vi "Process.vi"(8 "error in (no error)":errorcluster, 11 "DB2":refnum<class "DB2.lvclass">) -> (0 "error out":errorcluster, 3 "DB2 out":refnum<class "DB2.lvclass">)   [LabVIEW 2022 SP3, in "DB2.lvclass"]
uses:
  DB2.lvclass
  C:/Program Files (x86)/National Instruments/LabVIEW 2022/vi.lib/JKI/JKI SMO/SMO/SMO.lvclass
  <vilib>/JKI/JKI SMO/SMO/Typedefs/Parent Call--Enum.ctl
  Typedefs/PublicEvents--DB2.NewSettingsConfig.ctl
  <vilib>/JKI/JKI SMO/SMO/SMO.lvclass
  <vilib>/JKI/JKI SMO/SMO/SMO.lvclass/SMO.ctl
  <vilib>/JKI/JKI SMO/SMO/Private/GetVariant(Attr).vi
  <vilib>/JKI/JKI SMO/Support/Attribute.Identity/Read UniqueName.vi
  <vilib>/JKI/JKI SMO/Support/Attribute.Identity/Read Given Name.vi
  <vilib>/JKI/JKI SMO/Support/Attribute.Identity/Read ProspectiveOwner.vi
  <vilib>/JKI/JKI SMO/SMO/Private/ReftoDVR--SMO.vi
  <vilib>/JKI/JKI SMO/Support/Attribute.Identity/Attribute.Identity.lvclass
panel:
  in  "Cancel Button":bool
  in  "Save Button":bool
  in  "Source Code to Analyze":path
  in  "Report Generation Save Path":path
  in  "Requirements Definition (.csv)":path
  in  "OK":bool
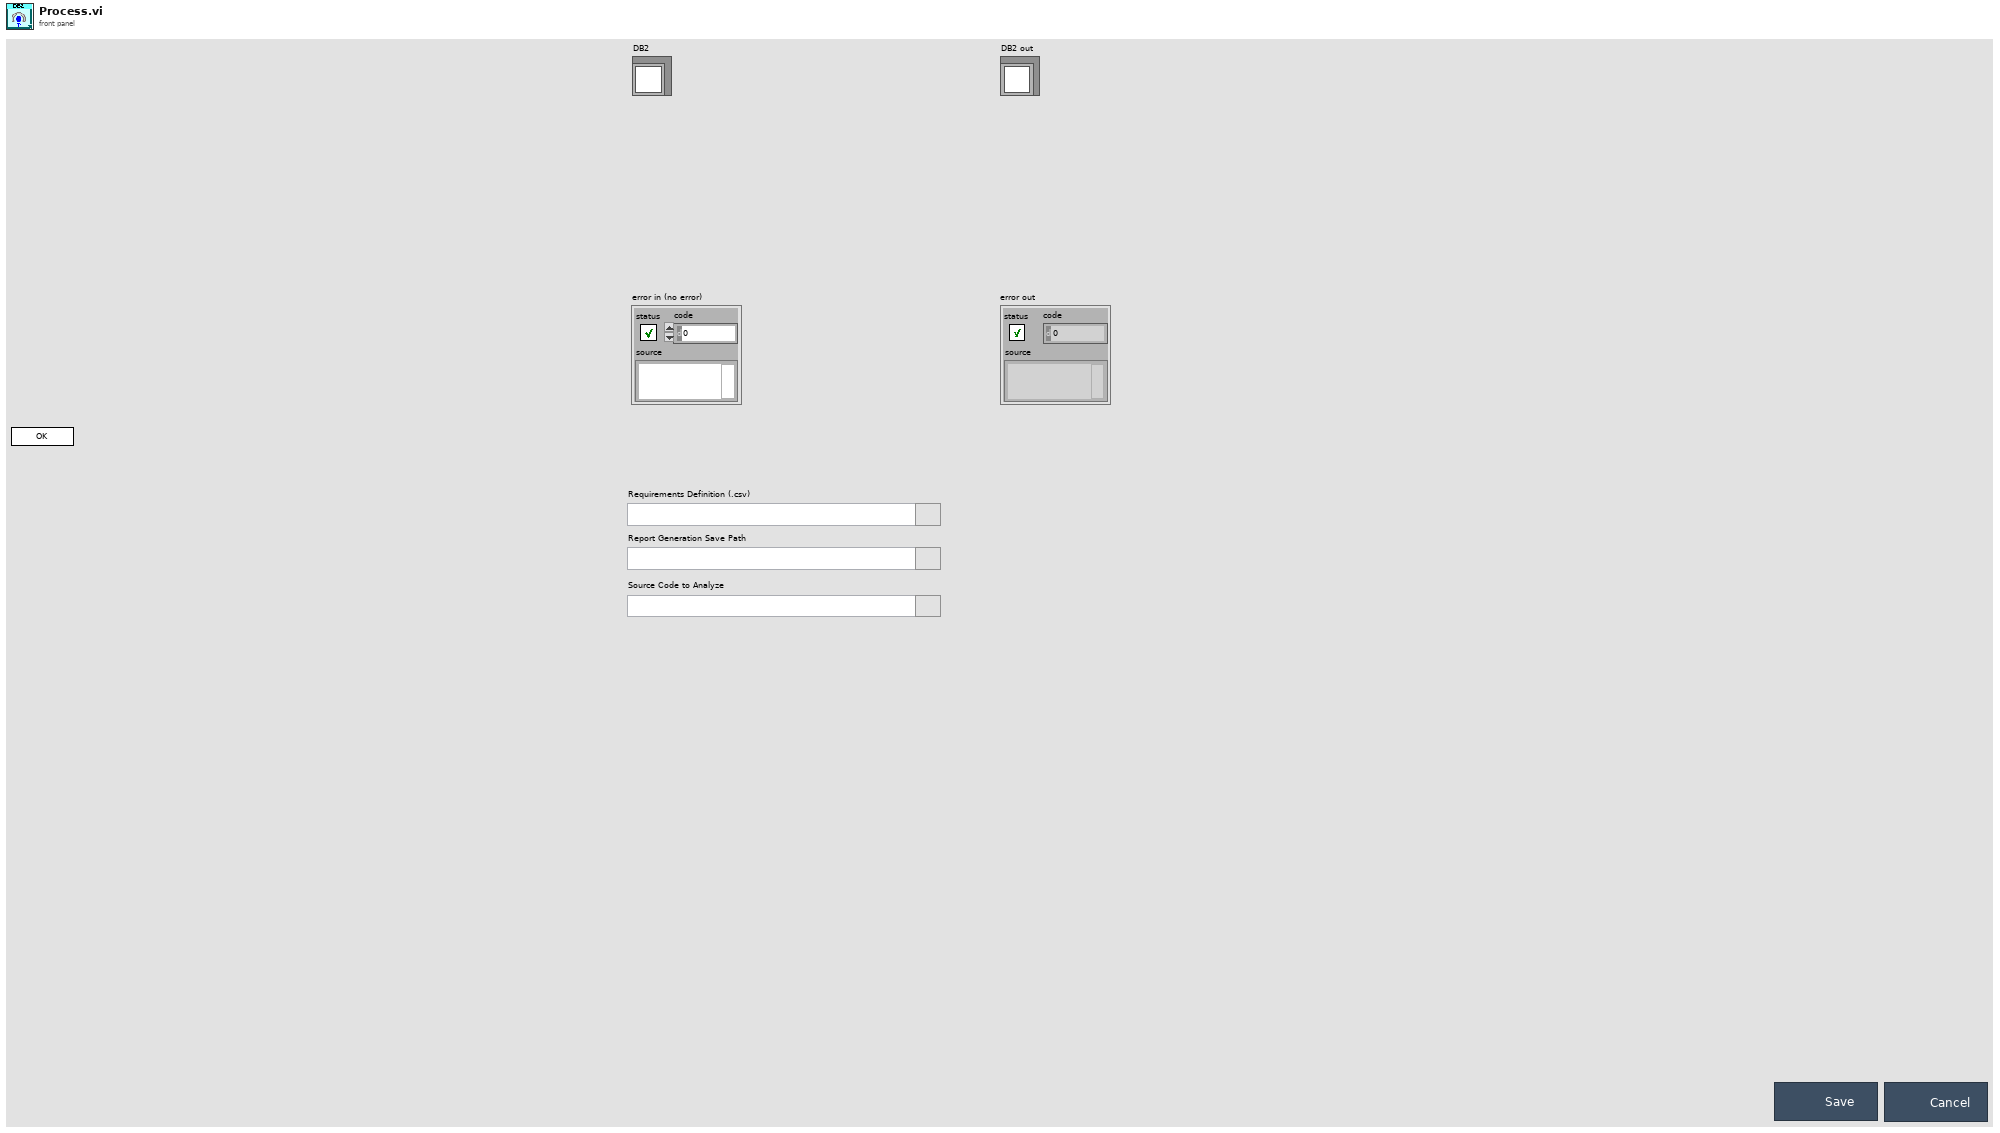
[diagram p1: front panel]
types:
  T1 = typedef "SMO.lvclass/Parent Call--Enum.ctl" = enum16{"Allows parent to run", "Does not request parent to run"}
  T2 = typedef "DB2.lvclass/PublicEvents--DB2.NewSettingsConfig.ctl" = cluster{"Requirements Definition (.csv)":path, "Report Generation Save Path":path, "Source Code to Analyze":path, "Search By:":string, "Word/Phrase:":string}
  T3 = enum32{"invalid app kind", "Development System", "Run Time System", "Student Edition", "Embedded LabVIEW", "Evaluation", "Custom"}
  T4 = enum32{"Invalid", "Standard", "Closed", "Hidden", "Minimized", "Maximized"}
  T5 = typedef "DB2.lvclass/DB2 State--enum.ctl" = enum16{"unknown", "Opened", "Embedded", "Closed"}
  T6 = cluster{"Core":cluster{"Current VI Reference":refnum<vi>, "Close Panel on Exit?":bool, "error":errorcluster}, "Self Ref":refnum<class "DB2.lvclass">, "New Settings Config":T2}
  T7 = cluster{"Current VI Reference":refnum<vi>, "Close Panel on Exit?":bool, "error":errorcluster}
  T8 = typedef "SMO.lvclass/Protected Events.ctl" = cluster{"StopProcesses":refnum<user-event>, "AbortProcesses":refnum<user-event>, "Config Changed":refnum<user-event>, "Dependency":refnum<user-event>}
  T9 = typedef "DB2.lvclass/PublicEvents--Cluster.ctl" = cluster{"UI State":refnum<user-event>, "NewSettingsConfig":refnum<user-event>}
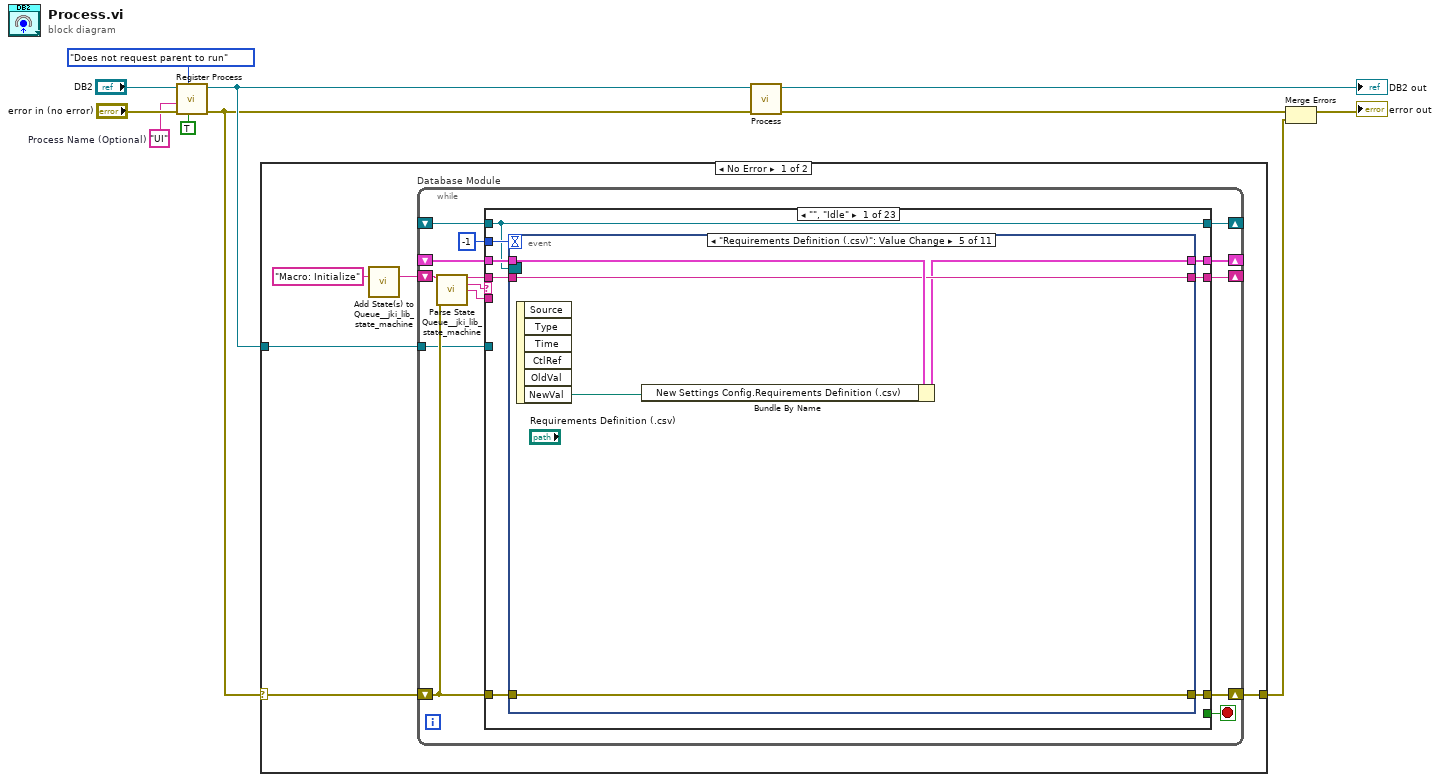
[diagram p0: block diagram]
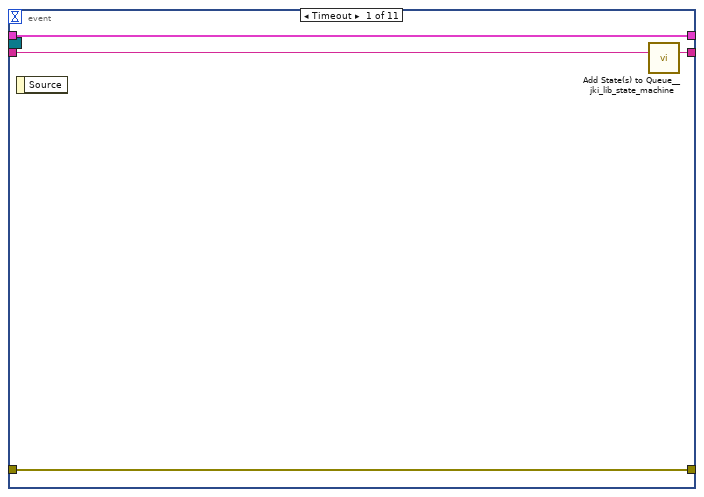
[diagram p2: hidden frame]
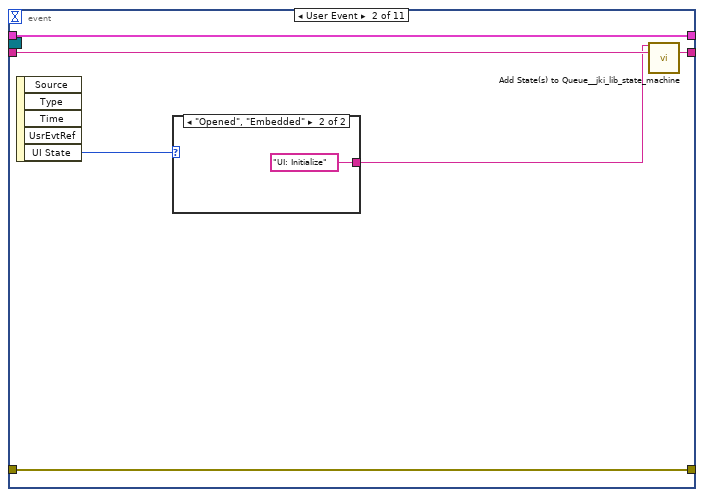
[diagram p3: hidden frame]
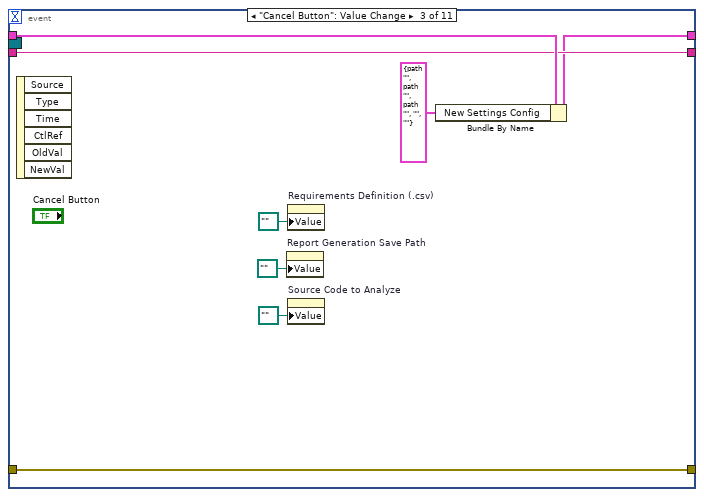
[diagram p5: hidden frame]
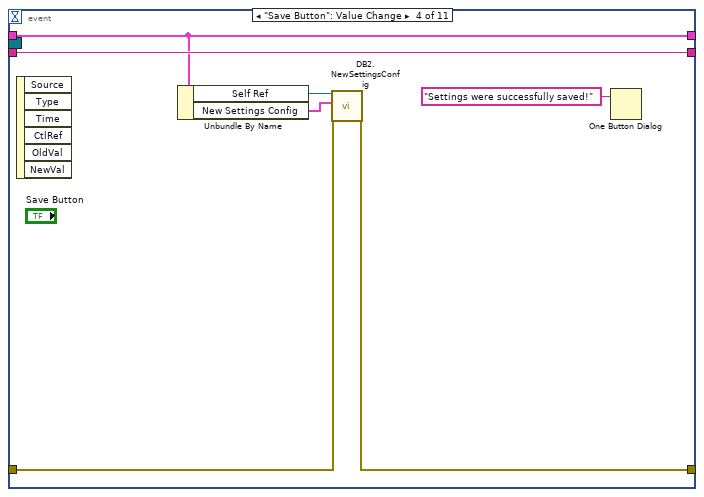
[diagram p6: hidden frame]
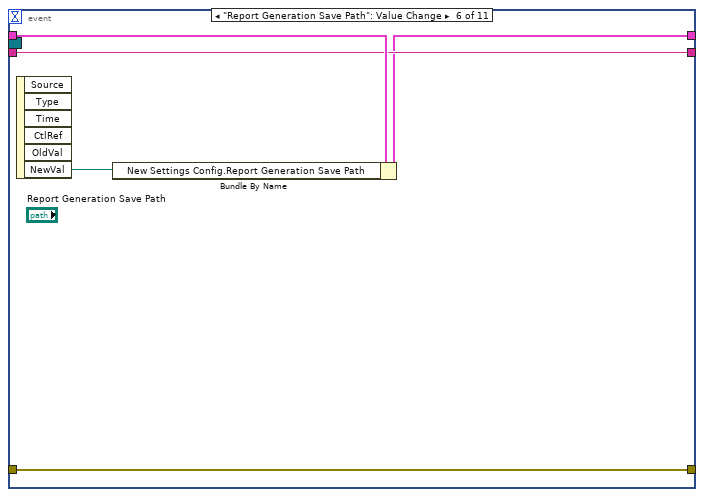
[diagram p7: hidden frame]
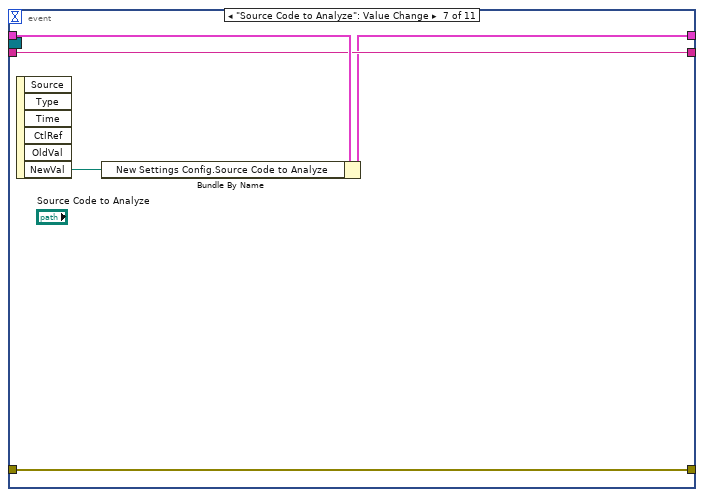
[diagram p8: hidden frame]
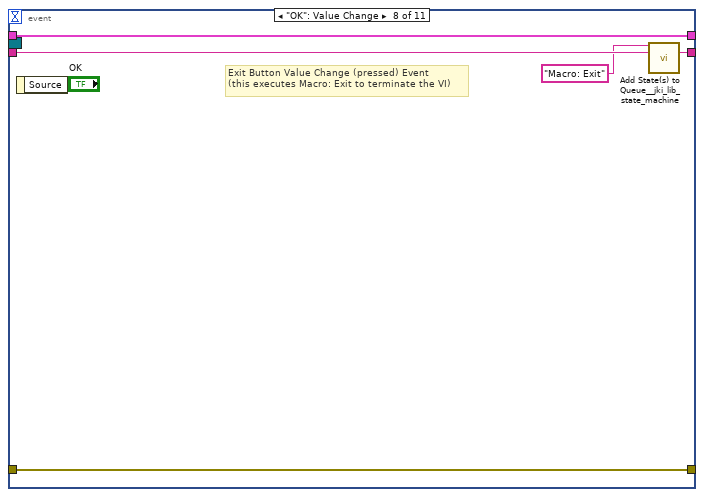
[diagram p9: hidden frame]
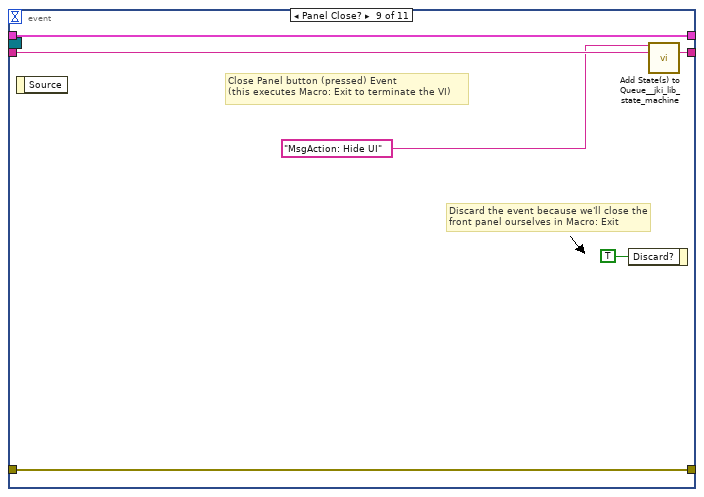
[diagram p10: hidden frame]
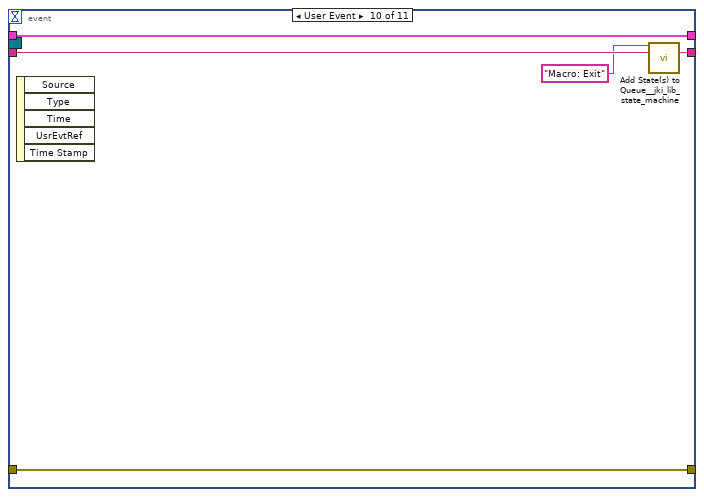
[diagram p11: hidden frame]
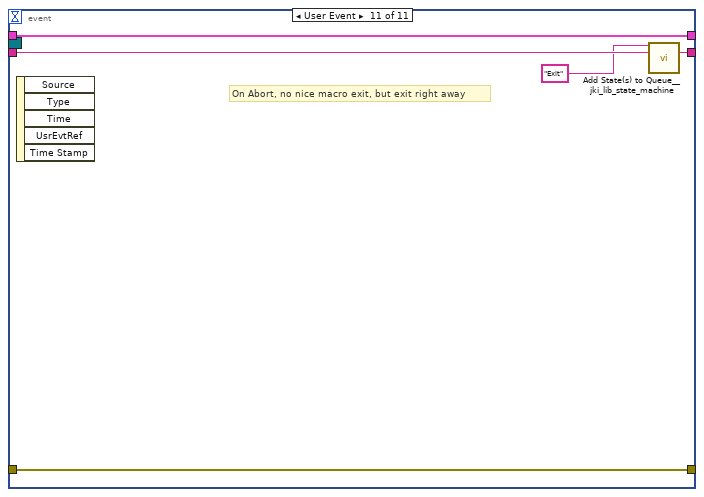
[diagram p12: hidden frame]
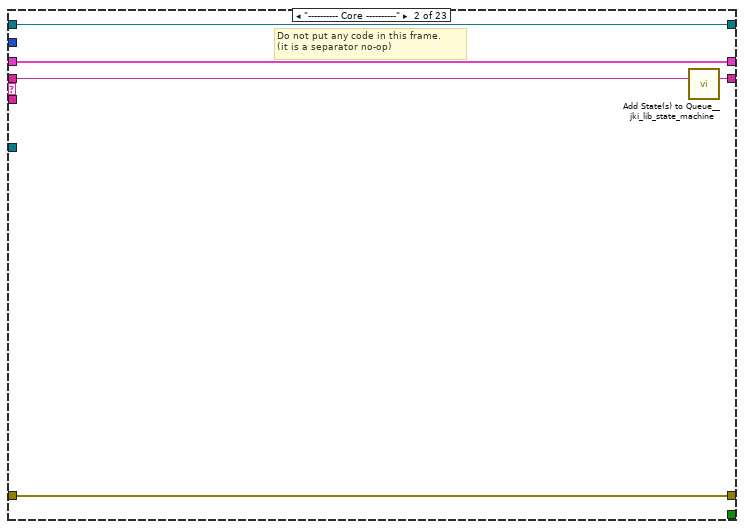
[diagram p13: hidden frame]
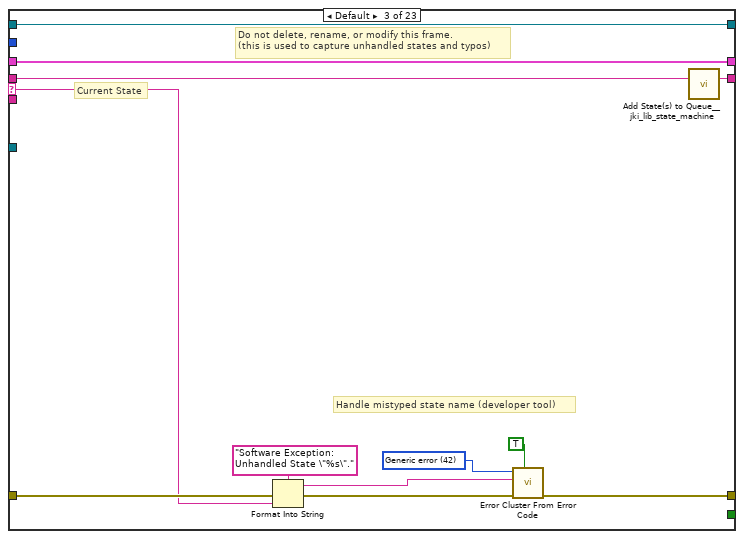
[diagram p14: hidden frame]
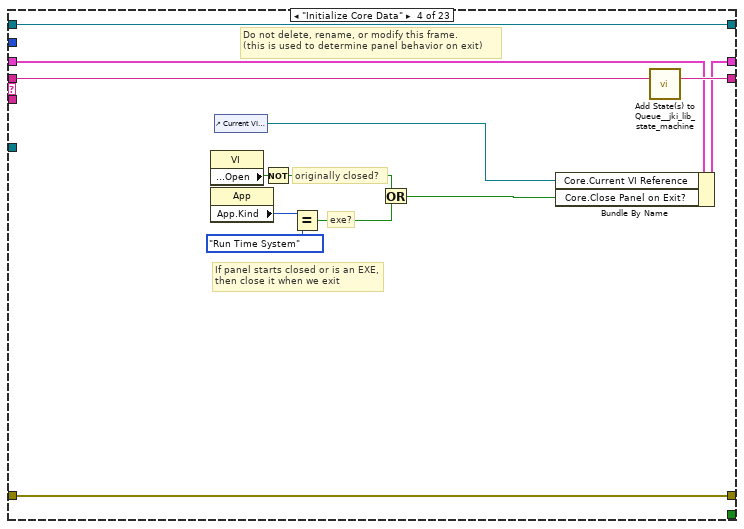
[diagram p15: hidden frame]
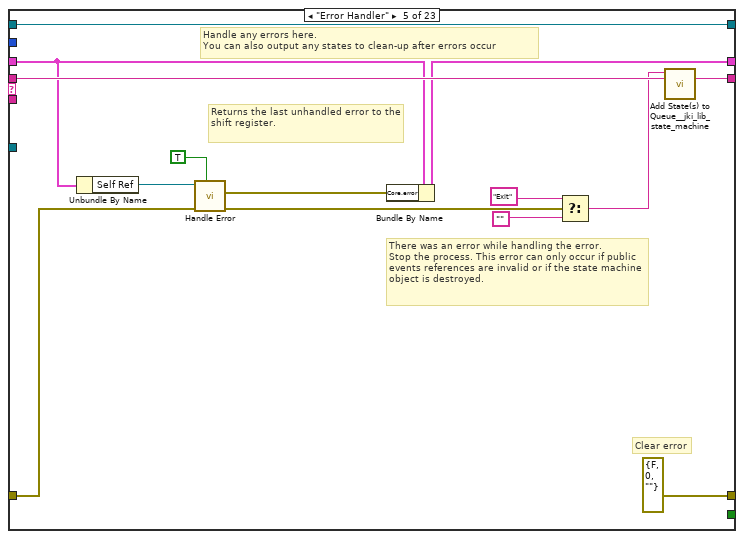
[diagram p16: hidden frame]
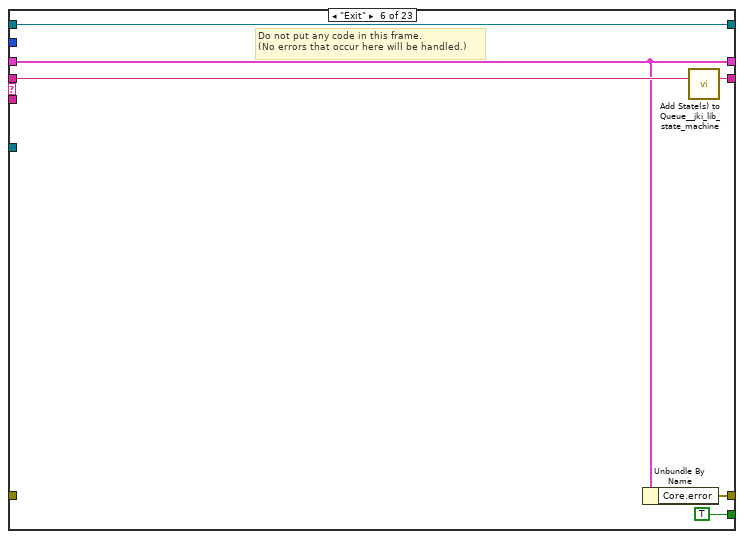
[diagram p17: hidden frame]
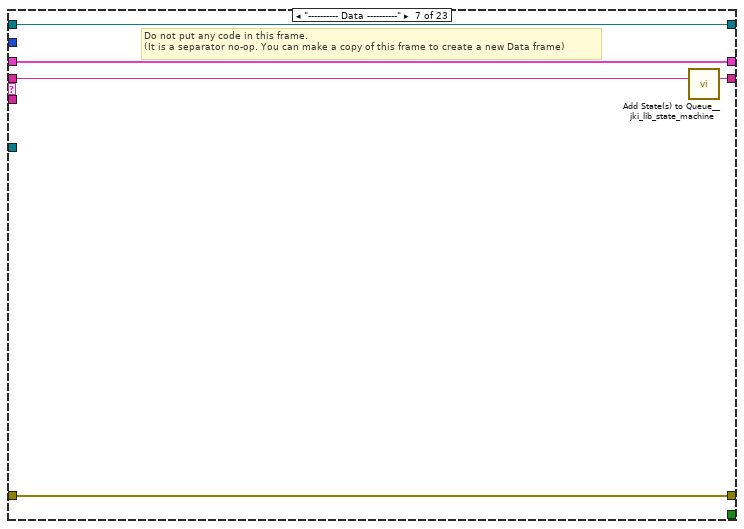
[diagram p18: hidden frame]
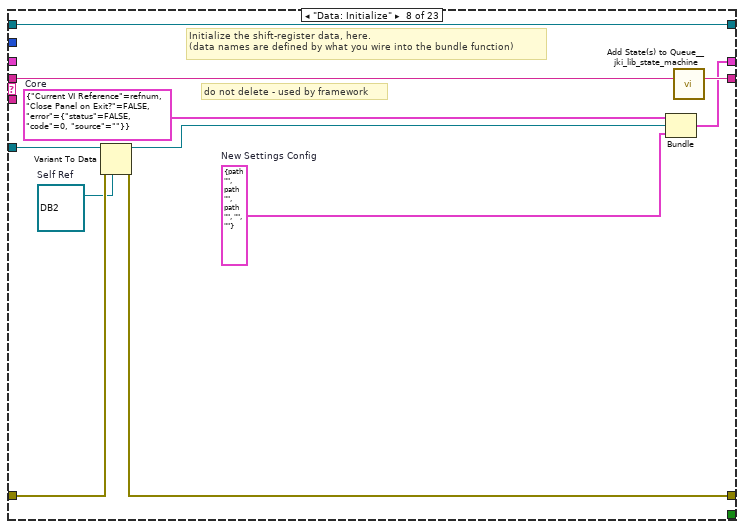
[diagram p19: hidden frame]
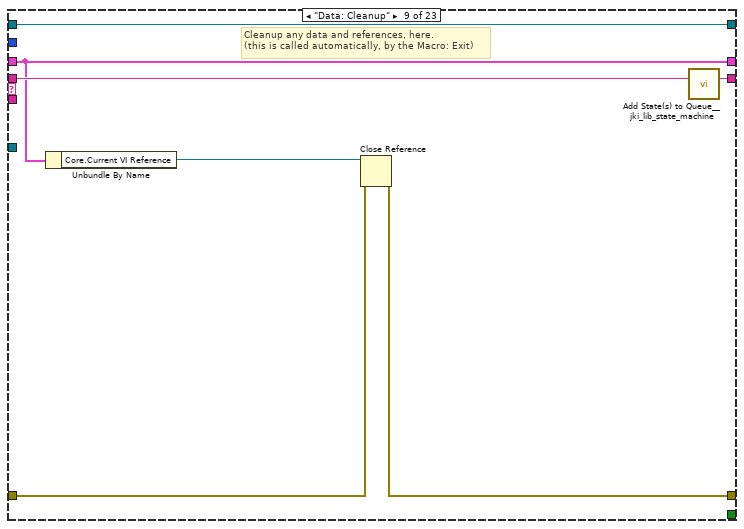
[diagram p20: hidden frame]
diagram:
  w4 = "UI"  # Process Name (Optional)
  n1 = call <vilib>:"Register Process.vi"("Forces Self to Run (F)"=TRUE, "Parent Call"=Parent_Call--Enum."Does not request parent to run", "error in (no error)"="error in (no error)", "Process Name (optional)"=w4, "SMO"="DB2") -> ("error out"=w10:errorcluster, "SMO out"=w11:refnum<class "DB2.lvclass">)  [unwired: 5 in]
  n2 = case shown="No Error" w10 {
    selector: w10 -> [w13 w318]
    tunnel: w11 -> [w14 _]
    tunnel: [w12 w318] -> w8
    frame No Error {
      n3 = call <vilib>:"Add State(s) to Queue__jki_lib_state_machine.vi"("State(s) in (\"\")"="Macro: Initialize") -> ("States Out"=w16:string)  [unwired: 14 in]
      n4 = while "Database Module" {
        shift-right: [w23] -> _
        shift-left: _ -> [w22]
        shift-right: [w26] -> w12
        shift-left: w13 -> [w20]
        shift-right: [w25] -> _
        shift-left: w16 -> [w27]
        tunnel: w14 -> [w19]
        shift-right: [w18] -> _
        shift-left: _ -> [w17]
        stop <- w24 stop-if-true
        n5 = call <vilib>:"Parse State Queue__jki_lib_state_machine.vi"("State Queue"=w27, "Error In (no error)"=w20) -> ("Remaining States"=w29:string, "Current State"=w30:string, "Arguments"=w28:string)  [unwired: 11 in]
        n6 = case shown="\"\", \"Idle\"" w30 {
          selector: w30 -> [_ _ w107 _ _ _ _ _ _ _ _ _ _ _ _ _ _ _ _ _ _ _ _]
          tunnel: w29 -> [w38 w105 w111 w130 w144 w150 w155 w166 w173 w178 w186 w193 w209 w241 w250 w261 w266 w277 w289 w294 w306 w312 w317]
          tunnel: w28 -> [_ _ _ _ _ _ _ _ _ _ _ w187 w205 _ _ _ _ _ _ _ _ _ _]
          tunnel: w22 -> [w36 w102 w109 w121 w140 w145 w152 _ w168 w175 w184 w191 w207 w238 w246 w252 w263 w274 w286 w291 w304 w310 w314]
          tunnel: [w35 w103 w113 w127 errorcluster {"status"=FALSE, "code"=0, "source"=""} ("error out") w146 w153 w158 w169 w176 w183 w188 w202 w239 w248 w259 w264 w268 w284 w292 w302 w308 w315] -> w26
          tunnel: w20 -> [w34 w103 w112 w127 w137 _ w153 w163 w170 w176 w183 w189 w203 w239 w248 w259 w264 w269 w281 w292 w295 w308 w315]
          tunnel: [w37 w104 w110 w129 w143 w149 w154 w165 w172 w177 w185 w192 w208 w240 w249 w260 w265 w276 w288 w293 w305 w311 w316] -> w25
          tunnel: [_ _ _ _ _ TRUE _ _ _ _ _ _ _ _ _ _ _ _ _ _ _ _ _] -> w24
          tunnel: [w33 w102 w109 w128 w139 w145 w152 w164 w168 w175 w184 w191 w207 w238 w246 w252 w263 w274 w286 w291 w304 w310 w314] -> w23
          tunnel: -1 ("Timeout") -> [w32 _ _ _ _ _ _ _ _ _ _ _ _ _ _ _ _ _ _ _ _ _ _]
          tunnel: w19 -> [_ _ _ _ _ _ _ w162 _ _ _ _ _ _ _ _ _ _ _ _ _ _ _]
          tunnel: [w31 w101 w106 w118 w142 w147 w151 w161 w167 w174 w182 w190 w206 w237 w247 w253 w262 w275 w287 w290 w301 w309 w313] -> w18
          tunnel: w17 -> [w31 w101 w106 w118 w142 w147 w151 w161 w167 w174 w182 w190 w206 w237 w247 w253 w262 w275 w287 w290 _ w309 w313]
          frame "", "Idle" {
            n7 = event shown="[4] \"Requirements Definition (.csv)\": Value Change" {
              selector: w31 -> [_ _ _ _ _ _ _ _ _ _ _]
              dyn-events: _ -> [_ _ _ _ _ _ _ _ _ _ _]
              timeout: w32 -> [_ _ _ _ _ _ _ _ _ _ _]
              tunnel: w38 -> [w42 w48 w56 w64 w68 w73 w78 w84 w90 w95 w100]
              tunnel: [w41 w47 w56 w64 w68 w73 w78 w83 w89 w94 w99] -> w37
              tunnel: w36 -> [w39 w45 w57 w63 w69 w74 w79 w81 w86 w92 w97]
              tunnel: [w40 w46 w55 w59 w67 w72 w77 w82 w88 w93 w98] -> w35
              tunnel: w34 -> [w40 w46 w55 w60 w67 w72 w77 w82 w88 w93 w98]
              tunnel: [w39 w45 w54 w63 w66 w71 w76 w81 w86 w92 w97] -> w33
              event Timeout {
                n8 = event-data() -> ()  [unwired: 1 in, 1 out]
                n9 = call <vilib>:"Add State(s) to Queue__jki_lib_state_machine.vi"("State(s) in (\"\")"=w42) -> ("States Out"=w41:string)  [unwired: 14 in]
              }
              event User Event {
                n10 = event-data() -> ("UI State"=w44:T5)  [unwired: 1 in, 4 out]
                n11 = case shown="\"Opened\", \"Embedded\"" w44 {
                  tunnel: [_ "UI: Initialize" ("State(s) in Front (\"\")")] -> w43
                  frame Default {
                  }
                  frame "Opened", "Embedded" {
                  }
                }
                n12 = call <vilib>:"Add State(s) to Queue__jki_lib_state_machine.vi"("State(s) in Front (\"\")"=w43, "State(s) in (\"\")"=w48) -> ("States Out"=w47:string)  [unwired: 13 in]
              }
              event "Cancel Button": Value Change {
                n13 = event-data() -> ()  [unwired: 1 in, 6 out]
                n14 = property on="Report Generation Save Path" class="Path"("Value"=path "" ("Report Generation Save Path")) -> ()  [unwired: 2 in, 2 out]
                n15 = property on="Requirements Definition (.csv)" class="Path"("Value"=path "" ("Requirements Definition (.csv)")) -> ()  [unwired: 2 in, 2 out]
                n16 = property on="Source Code to Analyze" class="Path"("Value"=path "" ("Source Code to Analyze")) -> ()  [unwired: 2 in, 2 out]
                n17 = Bundle By Name(cluster=w57, "New Settings Config"=T2 {"Requirements Definition (.csv)"=path "", "Report Generation Save Path"=path "", "Source Code to Analyze"=path "", "Search By:"="", "Word/Phrase:"=""}) -> (w54:T6)
              }
              event "Save Button": Value Change {
                n18 = event-data() -> ()  [unwired: 1 in, 6 out]
                n19 = Unbundle By Name(w63) -> ("Self Ref"=w62:refnum<class "DB2.lvclass">, "New Settings Config"=w61:T2)
                n20 = call "DB2.NewSettingsConfig.vi"("error in"=w60, "New Settings Config"=w61, "DB2.lvclass"=w62) -> ("error out"=w59:errorcluster)  [unwired: 7 in, 1 out]
                n21 = One Button Dialog(message="Settings were successfully saved!") -> ()  [unwired: 1 in, 1 out]
              }
              event "Requirements Definition (.csv)": Value Change {
                n22 = event-data() -> ("NewVal"=w65:path)  [unwired: 1 in, 5 out]
                n23 = Bundle By Name(cluster=w69, "New Settings Config.Requirements Definition (.csv)"=w65) -> (w66:T6)
              }
              event "Report Generation Save Path": Value Change {
                n24 = event-data() -> ("NewVal"=w70:path)  [unwired: 1 in, 5 out]
                n25 = Bundle By Name(cluster=w74, "New Settings Config.Report Generation Save Path"=w70) -> (w71:T6)
              }
              event "Source Code to Analyze": Value Change {
                n26 = event-data() -> ("NewVal"=w75:path)  [unwired: 1 in, 5 out]
                n27 = Bundle By Name(cluster=w79, "New Settings Config.Source Code to Analyze"=w75) -> (w76:T6)
              }
              event "OK": Value Change {
                # "Exit Button Value Change (pressed) Event\n(this executes Macro: Exit to terminate the VI)"
                n28 = event-data() -> ()  [unwired: 1 in, 1 out]
                n29 = call <vilib>:"Add State(s) to Queue__jki_lib_state_machine.vi"("State(s) in Front (\"\")"="Macro: Exit", "State(s) in (\"\")"=w84) -> ("States Out"=w83:string)  [unwired: 13 in]
              }
              event Panel Close? {
                # "Discard the event because we'll close the front panel ourselves in Macro: Exit"
                # "Close Panel button (pressed) Event\n(this executes Macro: Exit to terminate the VI)"
                n30 = event-data() -> ()  [unwired: 1 in, 1 out]
                n31 = event-data("Discard?"=TRUE) -> ()  [unwired: 1 in, 1 out]
                n32 = call <vilib>:"Add State(s) to Queue__jki_lib_state_machine.vi"("State(s) in Front (\"\")"="MsgAction: Hide UI", "State(s) in (\"\")"=w90) -> ("States Out"=w89:string)  [unwired: 13 in]
              }
              event User Event {
                n33 = event-data() -> ()  [unwired: 1 in, 5 out]
                n34 = call <vilib>:"Add State(s) to Queue__jki_lib_state_machine.vi"("State(s) in Front (\"\")"="Macro: Exit", "State(s) in (\"\")"=w95) -> ("States Out"=w94:string)  [unwired: 13 in]
              }
              event User Event {
                # "On Abort, no nice macro exit, but exit right away"
                n35 = event-data() -> ()  [unwired: 1 in, 5 out]
                n36 = call <vilib>:"Add State(s) to Queue__jki_lib_state_machine.vi"("State(s) in Front (\"\")"="Exit", "State(s) in (\"\")"=w100) -> ("States Out"=w99:string)  [unwired: 13 in]
              }
            }
          }
          frame "---------- Core ----------" {
            # "Do not put any code in this frame.\n(it is a separator no-op)"
            n37 = call <vilib>:"Add State(s) to Queue__jki_lib_state_machine.vi"("State(s) in (\"\")"=w105) -> ("States Out"=w104:string)  [unwired: 14 in]
          }
          frame Default {
            w116 = 42 items=["No error", "Argument error", "Memory is full", "Out of zone", "End of file", "File already open", "Generic file I/O error", "File not found", "File permission error", "Disk is full", "Duplicate path", "Too many files open", "System feature not enabled", "Resource file not found", "Cannot add resource", "Resource not found", "Image not found", "Image memory error", "Pen does not exist", "Config type invalid", "Config token not found", "Config parse error", "Config memory error", "Bad external code format", "Bad external code offset", "External code not present", "Null window", "Destroy window error", "Null menu", "Print aborted", "Bad print record", "Print driver error", "Windows error during printing", "Memory error during printing", "Print dialog error", "Generic print error", "Invalid device refnum", "Device not found", "Device parameter error", "Device unit error", "Cannot open device", "Device call aborted", "Generic error", "Cancelled by user", "Object ID too low", "Object ID too high", "Object not in heap", "Unknown heap", "Unknown object (invalid DefProc)", "Unknown object (DefProc not in table)", "Message out of range", "Invalid (null) method", "Unknown message", "Manager call not supported", "Bad address", "Network operation in progress", "Network operation timed out", "Connection is busy", "Network attribute not supported", "Network error", "Address in use", "System out of memory", "Connection aborted", "Connection refused", "Not connected", "Already connected", "Connection closed", "Initialization error (interapplication manager)", "Bad occurrence", "Wait on unbound occurrence handler", "Occurrence queue overflow", "Datalog type conflict", "Unused", "Unrecognized type (interapplication manager)", "Memory corrupt", "Failed to make temporary DLL", "Old CIN version", "Drag socket not found", "Failed to load drop-object", "Failed to register OLE object", "Failed to release OLE object", "Format specifier type mismatch", "Unknown format specifier", "Too few format specifiers", "Too many format specifiers", "Scan failed", "Newer CIN version", "Error converting to variant", "Runtime menu error", "Password tampered", "Variant attribute not found", "Incompatible variant data type", "Event data is not available", "Event Store is not present", "Occurrence is not found", "Event Queue is not created", "Event info is not available", "Refnum passed is NULL", "Error retrieving Class GUID", "Error retrieving CoClass GUID", "Error retrieving TypeLib GUID.", "Bad built application magic bytes.", "Specific driver is different from the specific driver associated with the Logical Name.", "There is no session opened to the class driver.", "Max Error", "MAX - Error with config objects", "MAX - Error loading configuration", "MAX - Group not supported"]
            # "Current State"
            # "Do not delete, rename, or modify this frame.\n(this is used to capture unhandled states and typos)"
            # "Handle mistyped state name (developer tool)"
            n38 = Format Into String(format string="Software Exception: Unhandled State \"%s\"." ("message"), error in=w112, w107) -> (resulting string=w115:string, error out=w114:errorcluster)  [unwired: 1 in]
            n39 = call <vilib>:"Error Cluster From Error Code.vi"("show call chain? (False)"=TRUE, "error in (no error)"=w114, "error message (\"\")"=w115, "error code (0)"=w116) -> ("error out"=w113:errorcluster)  [unwired: 5 in]
            n40 = call <vilib>:"Add State(s) to Queue__jki_lib_state_machine.vi"("State(s) in (\"\")"=w111) -> ("States Out"=w110:string)  [unwired: 14 in]
          }
          frame "Initialize Core Data" {
            # "Do not delete, rename, or modify this frame.\n(this is used to determine panel behavior on exit)"
            # "originally closed?"
            # "exe?"
            # "If panel starts closed or is an EXE, then close it when we exit"
            n41 = property class="VI"() -> ("Front Panel.Open"=w126:bool)  [unwired: 2 in, 2 out]
            n42 = property class="App"() -> ("App.Kind"=w125:T3)  [unwired: 2 in, 2 out]
            n43 = control-ref of="Current VI Reference"() -> (w119:refnum<vi>)
            n44 = Not(x=w126) -> (.not. x?=w123:bool)
            n45 = Equal?(x=w125, y=T3."Run Time System" ("Application:Kind")) -> (x = y?=w122:bool)
            n46 = Or(x=w123, y=w122) -> (x .or. y?=w120:bool)
            n47 = Bundle By Name(cluster=w121, "Core.Current VI Reference"=w119, "Core.Close Panel on Exit?"=w120) -> (w128:T6)
            n48 = call <vilib>:"Add State(s) to Queue__jki_lib_state_machine.vi"("State(s) in (\"\")"=w130) -> ("States Out"=w129:string)  [unwired: 14 in]
          }
          frame "Error Handler" {
            # "Returns the last unhandled error to the shift register."
            # "There was an error while handling the error.\nStop the process. This error can only occur if public events references are invalid or if the state machine object is destroyed."
            # "Handle any errors here.\nYou can also output any states to clean-up after errors occur"
            # "Clear error"
            n49 = Unbundle By Name(w140) -> ("Self Ref"=w141:refnum<class "DB2.lvclass">)
            n50 = call-dynamic "Handle Error.vi"("Stop on Unhandled Error (T)"=TRUE, "error in"=w137, "SMO"=w141) -> ("handling error"=w135:errorcluster, "Unhandled error"=w138:errorcluster)  [unwired: 6 in, 1 out]
            n51 = Bundle By Name(cluster=w140, "Core.error"=w138) -> (w139:T6)
            n52 = Select(t="Exit", s=w135, f="") -> (s? t:f=w132:string)
            n53 = call <vilib>:"Add State(s) to Queue__jki_lib_state_machine.vi"("State(s) in Front (\"\")"=w132, "State(s) in (\"\")"=w144) -> ("States Out"=w143:string)  [unwired: 13 in]
          }
          frame "Exit" {
            # "Do not put any code in this frame.\n(No errors that occur here will be handled.)"
            n54 = Unbundle By Name(w145) -> ("Core.error"=w146:errorcluster)
            n55 = call <vilib>:"Add State(s) to Queue__jki_lib_state_machine.vi"("State(s) in (\"\")"=w150) -> ("States Out"=w149:string)  [unwired: 14 in]
          }
          frame "---------- Data ----------" {
            # "Do not put any code in this frame.\n(It is a separator no-op. You can make a copy of this frame to create a new Data frame)"
            n56 = call <vilib>:"Add State(s) to Queue__jki_lib_state_machine.vi"("State(s) in (\"\")"=w155) -> ("States Out"=w154:string)  [unwired: 14 in]
          }
          frame "Data: Initialize" {
            w156 = T2 {"Requirements Definition (.csv)"=path "", "Report Generation Save Path"=path "", "Source Code to Analyze"=path "", "Search By:"="", "Word/Phrase:"=""}  # New Settings Config
            w157 = T7 {"Current VI Reference"=refnum, "Close Panel on Exit?"=FALSE, "error"={"status"=FALSE, "code"=0, "source"=""}}  # Core
            w160 = refnum<class "DB2.lvclass"> refnum  # Self Ref
            # "do not delete - used by framework"
            # "Initialize the shift-register data, here.\n(data names are defined by what you wire into the bundle function)"
            n57 = Variant To Data(error in=w163, type=w160, Variant=w162) -> (data=w159:refnum<class "DB2.lvclass">, error out=w158:errorcluster)
            n58 = Bundle("Core"=w157, "Self Ref"=w159, "New Settings Config"=w156) -> (w164:T6)  [unwired: 1 in]
            n59 = call <vilib>:"Add State(s) to Queue__jki_lib_state_machine.vi"("State(s) in (\"\")"=w166) -> ("States Out"=w165:string)  [unwired: 14 in]
          }
          frame "Data: Cleanup" {
            # "Cleanup any data and references, here.\n(this is called automatically, by the Macro: Exit)"
            n60 = Unbundle By Name(w168) -> ("Core.Current VI Reference"=w171:refnum<vi>)
            n61 = Close Reference(reference=w171, error in (no error)=w170) -> (error out=w169:errorcluster)
            n62 = call <vilib>:"Add State(s) to Queue__jki_lib_state_machine.vi"("State(s) in (\"\")"=w173) -> ("States Out"=w172:string)  [unwired: 14 in]
          }
          frame "---------- UI ----------" {
            # "Do not put any code in this frame.\n(It is a separator no-op. You can make a copy of this frame to create a new UI frame)"
            n63 = call <vilib>:"Add State(s) to Queue__jki_lib_state_machine.vi"("State(s) in (\"\")"=w178) -> ("States Out"=w177:string)  [unwired: 14 in]
          }
          frame "UI: Initialize" {
            n64 = property on="Report Generation Save Path" class="Path"("Value"=path "" ("Report Generation Save Path")) -> ()  [unwired: 2 in, 2 out]
            n65 = property on="Requirements Definition (.csv)" class="Path"("Value"=path "" ("Requirements Definition (.csv)")) -> ()  [unwired: 2 in, 2 out]
            n66 = property on="Source Code to Analyze" class="Path"("Value"=path "" ("Source Code to Analyze")) -> ()  [unwired: 2 in, 2 out]
            n67 = call <vilib>:"Add State(s) to Queue__jki_lib_state_machine.vi"("State(s) in (\"\")"=w186) -> ("States Out"=w185:string)  [unwired: 14 in]
          }
          frame "UI: Cursor Set" {
            # "Argument"
            # "Initialize the User Interface, here.\n(this is called automatically, by the Macro: Init)"
            n68 = disable-structure shown="Default" {
              disable-tunnel: w189 -> [w194 w197]
              disable-tunnel: [w194 w196] -> w188
              disable-tunnel: w187 -> [_ w195]
              frame condition #0 {
              }
              frame condition #1 (active) {
                n69 = case shown="\"Idle\", Default" w195 {
                  tunnel: w197 -> [w199 w201]
                  tunnel: [w198 w200] -> w196
                  frame "Idle", Default {
                    n70 = call <vilib>:"Unset Busy.vi"("error in (no error)"=w199) -> ("error out"=w198:errorcluster)  [unwired: 10 in]
                  }
                  frame "Busy" {
                    n71 = call <vilib>:"Set Busy.vi"("error in (no error)"=w201) -> ("error out"=w200:errorcluster)  [unwired: 9 in, 1 out]
                  }
                }
              }
            }
            n72 = call <vilib>:"Add State(s) to Queue__jki_lib_state_machine.vi"("State(s) in (\"\")"=w193) -> ("States Out"=w192:string)  [unwired: 14 in]
          }
          frame "UI: Front Panel State" {
            # "Argument"
            # "Set Front Panel Open or Closed\n(Usage: \"UI: Front Panel State >> Open|Close\")"
            n73 = Unbundle By Name(w207) -> ("Core.Current VI Reference"=w204:refnum<vi>)
            n74 = disable-structure shown="Default" {
              disable-tunnel: w203 -> [w213 w236]
              disable-tunnel: [w212 w236] -> w202
              disable-tunnel: w204 -> [w211 _]
              disable-tunnel: w205 -> [w210 _]
              frame condition #0 (active) {
                n75 = case shown="\"Open\"" w210 {
                  tunnel: w213 -> [w217 w230]
                  tunnel: [w219 w231] -> w212
                  tunnel: w211 -> [w218 w228]
                  frame "Open" {
                    # "Open FP if not open or invalid"
                    n76 = property class="VI"(reference=w218, error in=w217) -> (reference out=w215:refnum<vi>, error out=w216:errorcluster, "FP.State"=w214:T4)
                    n77 = case shown="Default" w214 {
                      tunnel: [w222 w225] -> w219
                      tunnel: w216 -> [w221 w225]
                      tunnel: w215 -> [w220 _]
                      frame Default {
                        n78 = invoke class="VI" method="FP.Open"(reference=w220, error in=w221, "Activate"=TRUE, "State"=T4."Standard") -> (error out=w222:errorcluster)  [unwired: 1 in, 4 out]
                      }
                      frame "Invalid", "Standard" {
                      }
                    }
                  }
                  frame "Close", Default {
                    # "Close FP is not Closed or Invalid"
                    n79 = property class="VI"(reference=w228, error in=w230) -> (reference out=w227:refnum<vi>, error out=w229:errorcluster, "FP.State"=w226:T4)
                    n80 = case shown="Default" w226 {
                      tunnel: [w232 w235] -> w231
                      tunnel: w229 -> [w232 w234]
                      tunnel: w227 -> [_ w233]
                      frame "Invalid", "Closed" {
                      }
                      frame Default {
                        n81 = invoke class="VI" method="FP.Close"(reference=w233, error in=w234) -> (error out=w235:errorcluster)  [unwired: 1 in, 2 out]
                      }
                    }
                  }
                }
              }
              frame condition #1 {
              }
            }
            n82 = call <vilib>:"Add State(s) to Queue__jki_lib_state_machine.vi"("State(s) in (\"\")"=w209) -> ("States Out"=w208:string)  [unwired: 14 in]
          }
          frame "---------- Macro ----------" {
            # "Do not put any code in this frame.\n(It is a separator no-op. You can make a copy of this frame to create a new Macro frame)"
            n83 = call <vilib>:"Add State(s) to Queue__jki_lib_state_machine.vi"("State(s) in (\"\")"=w241) -> ("States Out"=w240:string)  [unwired: 14 in]
          }
          frame "Macro: Initialize" {
            w244 = "UI: Initialize\n//UI: Front Panel State >> Open\n\n//Test: Start SMO Dependency //Only for development purpose."  # UI: Initialize //UI: Front Panel State >> Open  //Test: Start SMO Dependency //Only for development purpose.
            # "Initialization Macro\n(This is called once, when the VI starts)"
            n84 = call <vilib>:"Add State(s) to Queue__jki_lib_state_machine.vi"("State(s) in Front (\"\")"="Data: Initialize\nInitialize Core Data\nEvents: Register", "State(s) in (\"\")"="Process: Sync", "State(s) at Back (\"\")"=w244) -> ("States Out"=w243:string)  [unwired: 12 in]
            n85 = call <vilib>:"Add State(s) to Queue__jki_lib_state_machine.vi"("State(s) in Front (\"\")"=w243, "State(s) in (\"\")"=w250) -> ("States Out"=w249:string)  [unwired: 13 in]
          }
          frame "Macro: Exit" {
            # "Exit Macro\n(This is called once, when the VI exits)"
            n86 = Unbundle By Name(w252) -> ("Core.Close Panel on Exit?"=w258:bool)
            n87 = Select(t="UI: Front Panel State >> Close", s=w258, f="") -> (s? t:f=w255:string)
            n88 = call <vilib>:"Add State(s) to Queue__jki_lib_state_machine.vi"("State(s) in (\"\")"=w255, "State(s) at Back (\"\")"="Data: Cleanup\nEvents: Unregister\nProcess: Sync\nExit") -> ("States Out"=w254:string)  [unwired: 13 in]
            n89 = call <vilib>:"Add State(s) to Queue__jki_lib_state_machine.vi"("State(s) in Front (\"\")"=w254, "State(s) in (\"\")"=w261) -> ("States Out"=w260:string)  [unwired: 13 in]
          }
          frame "---------- Process ----------" {
            # "Template Separator\n(You can make a copy of, or modify, this frame)"
            n90 = call <vilib>:"Add State(s) to Queue__jki_lib_state_machine.vi"("State(s) in (\"\")"=w266) -> ("States Out"=w265:string)  [unwired: 14 in]
          }
          frame "Process: Sync" {
            n91 = Unbundle By Name(w274) -> ("Self Ref"=w270:refnum<class "DB2.lvclass">)
            n92 = call <vilib>:"WaitOnProcessSync.vi"("error in (no error)"=w269, "SMO"=w270) -> ("error out"=w268:errorcluster, "Don't run?"=w273:bool)  [unwired: 7 in, 1 out]
            n93 = Select(t="Data: Cleanup\nEvents: Unregister\nExit", s=w273, f="") -> (s? t:f=w267:string)
            n94 = call <vilib>:"Add State(s) to Queue__jki_lib_state_machine.vi"("State(s) in Front (\"\")"=w267, "State(s) in (\"\")"=w277) -> ("States Out"=w276:string)  [unwired: 13 in]
          }
          frame "Test: Start SMO Dependency" {
            # ">> Returns the instance of \"Dummy\"\nand ignores the other levels dependencies"
            n95 = Unbundle By Name(w286) -> ("Self Ref"=w285:refnum<class "DB2.lvclass">)
            n96 = call <vilib>:"LaunchDependency.vi"("error in (no error)"=w281, "Dependency Name"="Dummy", "Dependency Type"=refnum<class "SMO.lvclass"> refnum ("SMO.lvclass"), "SMO in"=w285) -> ("error out"=w284:errorcluster, "SMO out"=w278:refnum<class "DB2.lvclass">)  [unwired: 4 in, 2 out]
            n97 = call <vilib>:"ListThisLevelDependencies.vi"("SMO in"=w278) -> ("[My Dependencies]"=w280:refnum<class "SMO.lvclass">[])  [unwired: 8 in, 2 out]
            n98 = Index Array(array=w280) -> (element=w279:refnum<class "SMO.lvclass">)  [unwired: 1 in]
            n99 = call <vilib>:"Get Name.vi"("SMO"=w279) -> ()  [unwired: 6 in, 5 out]
            n100 = call <vilib>:"Add State(s) to Queue__jki_lib_state_machine.vi"("State(s) in (\"\")"=w289) -> ("States Out"=w288:string)  [unwired: 14 in]
          }
          frame "---------- Events ----------" {
            # "Template Separator\n(You can make a copy of, or modify, this frame)"
            n101 = call <vilib>:"Add State(s) to Queue__jki_lib_state_machine.vi"("State(s) in (\"\")"=w294) -> ("States Out"=w293:string)  [unwired: 14 in]
          }
          frame "Events: Register" {
            n102 = Unbundle By Name(w304) -> ("Self Ref"=w300:refnum<class "DB2.lvclass">)
            n103 = call <vilib>:"GetProtectedEvents.vi"("error in (no error)"=w295, "SMO"=w300) -> ("error out"=w296:errorcluster, "SMO Protected Events"=w303:T8, "SMO out"=w297:refnum<class "DB2.lvclass">)  [unwired: 7 in]
            n104 = call "DB2.GetPublicEvents.vi"("error in (no error)"=w296, "DB2"=w297) -> ("error out"=w298:errorcluster, "SMO.DB2 Public Events"=w299:T9)  [unwired: 7 in, 1 out]
            n105 = register-events(error in=w298, w303, w299) -> (reference out=w301:refnum<event-registration>, error out=w302:errorcluster)  [unwired: 1 in]
            n106 = call <vilib>:"Add State(s) to Queue__jki_lib_state_machine.vi"("State(s) in (\"\")"=w306) -> ("States Out"=w305:string)  [unwired: 14 in]
          }
          frame "Events: Unregister" {
            # "Your code here.\n(You can make a copy of, or modify, this frame)"
            n107 = Unregister For Events(event registration refnum=w309, error in=w308) -> (error out=w307:errorcluster)
            n108 = call <vilib>:"Clear Errors.vi"("error in (no error)"=w307) -> ()  [unwired: 5 in, 2 out]
            n109 = call <vilib>:"Add State(s) to Queue__jki_lib_state_machine.vi"("State(s) in (\"\")"=w312) -> ("States Out"=w311:string)  [unwired: 14 in]
          }
          frame "---------MsgAction---------" {
            # "MsgAction Separator\n(You can make a copy of, or modify, this frame)"
            n110 = call <vilib>:"Add State(s) to Queue__jki_lib_state_machine.vi"("State(s) in (\"\")"=w317) -> ("States Out"=w316:string)  [unwired: 14 in]
          }
        }
      }
    }
    frame Error {
    }
  }
  n111 = call-parent "Process.vi"("error in"=w10, "SMO"=w11) -> ("error out"=w9:errorcluster, "SMO out"=→"DB2 out":refnum<class "DB2.lvclass">)  [unwired: 8 in]
  n112 = Merge Errors(w9, w8) -> (→"error out":errorcluster)
